vi "Create Folder.vi"(8 "에러 입력":errorcluster caption="에러 입력(에러 없음)", 11 "폴더경로":path) -> (0 "error out":errorcluster caption="에러 출력", 3 "dup path":path)   [LabVIEW 2020]
uses:
  <vilib>/Utility/error.llb/Error Cluster From Error Code.vi
  <vilib>/ErrorRing/Error Ring.xnode
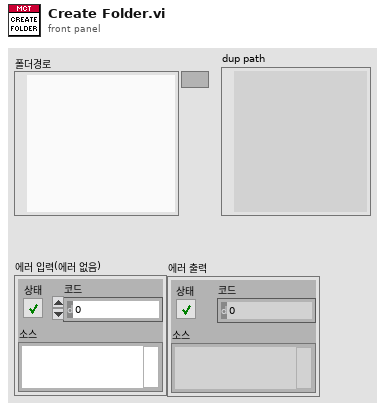
[diagram p1: front panel]
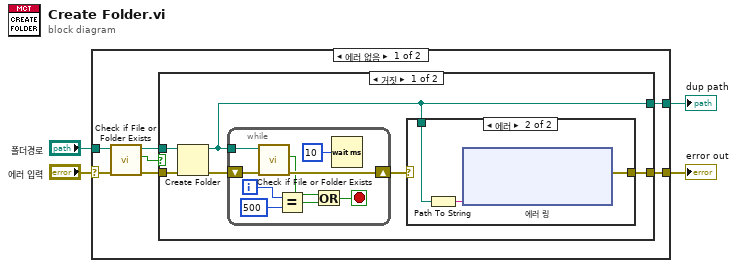
[diagram p0: block diagram]
diagram:
  n1 = case shown="에러 없음" "에러 입력" {
    selector: "에러 입력" -> [w7 w40]
    tunnel: "폴더경로" -> [w9 w41]
    tunnel: [w8 w40] -> w3
    tunnel: [w6 w41] -> w2
    frame No Error {
      n2 = call <vilib>:"Check if File or Folder Exists.vi"("error in (no error)"=w7, "path"=w9) -> ("error out"=w11:errorcluster, "file or folder exists?"=w5:bool, "dup path"=w10:path)  [unwired: 7 in]
      n3 = case shown="거짓" w5 {
        tunnel: w11 -> [w17 w39]
        tunnel: w10 -> [w16 w38]
        tunnel: [w15 w39] -> w8
        tunnel: [w13 w38] -> w6
        frame False {
          n4 = Create Folder(path (use dialog)=w16, error in=w17) -> (created path=w13:path, error out=w14:errorcluster)  [unwired: 1 in, 1 out]
          n5 = while {
            shift-right: [w25] -> w12
            shift-left: w14 -> [w26]
            tunnel: w13 -> [w24]
            i -> [w20]
            stop <- w22 stop-if-true
            n6 = call <vilib>:"Check if File or Folder Exists.vi"("error in (no error)"=w26, "path"=w24) -> ("error out"=w25:errorcluster, "file or folder exists?"=w23:bool)  [unwired: 7 in, 1 out]
            n7 = Equal?(x=w20, y=500) -> (x = y?=w21:bool)
            n8 = Or(x=w23, y=w21) -> (x .or. y?=w22:bool)
            n9 = Wait (ms)(milliseconds to wait=u32 10 ("대기 시간(ms)")) -> ()  [unwired: 1 out]
          }
          n10 = case shown="에러" w12 {
            selector: w12 -> [w27 _]
            tunnel: [w27 w30] -> w15
            tunnel: w13 -> [_ w29]
            frame No Error {
            }
            frame Error {
              n11 = Path To String(path=w29) -> (string=w28:string)
              n12 = xnode "에러 링"("파라미터 0"=w28) -> ("에러 출력"=w30:errorcluster)
            }
          }
        }
        frame True {
        }
      }
    }
    frame Error {
    }
  }
  "dup path" <- w2
  "error out" <- w3
